vi "CALC_Phi_theta_etc_3_(online).vi"(2 "Current frame #":u32, 3 "Twisted neck":bool, 4 "Use alternative magnets orientation":bool, 5 "Bridge swap":bool, 6 "SB size":u8, 7 "Input cluster of data":T1) -> (1 "Animal coordinates":T2)   [LabVIEW 2018, in "Tracker.lvlib"]
uses:
  Tracker.lvlib
  Controls/CTL_Animal_Coordinates_and_Speed.ctl
  Controls/CTL_Cage_Coords.ctl
  <vilib>/ptbypt/NI_PtbyPt.lvlib
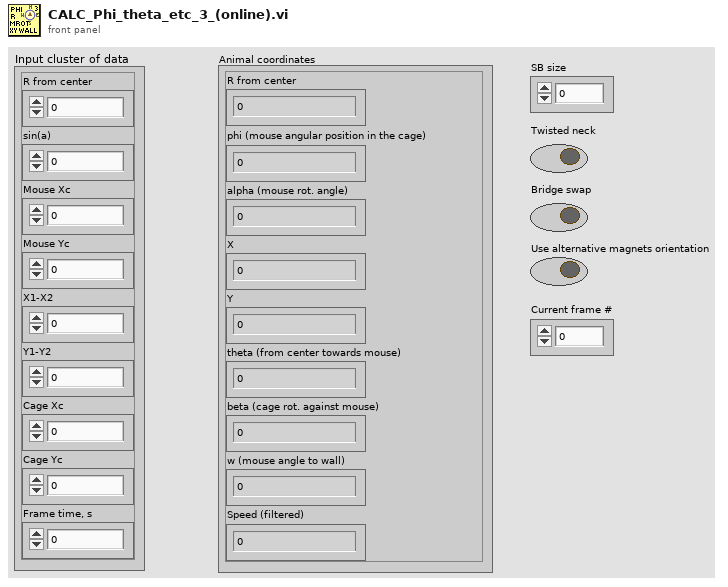
[diagram p1: front panel]
types:
  T1 = typedef "Tracker.lvlib/CTL_Cage_Coords.ctl" = cluster{"R from center":dbl, "sin(a)":dbl, "Mouse Xc":dbl, "Mouse Yc":dbl, "X1-X2":dbl, "Y1-Y2":dbl, "Cage Xc":dbl, "Cage Yc":dbl, "Frame time, s":dbl}
  T2 = typedef "Tracker.lvlib/CTL_Animal_Coordinates_and_Speed.ctl" = cluster{"R from center":dbl, "phi (mouse angular position in the cage)":dbl, "alpha (mouse rot. angle)":dbl, "X":dbl, "Y":dbl, "theta (from center towards mouse)":dbl, "beta (cage rot. against mouse)":dbl, "w (mouse angle to wall)":dbl, "Speed (filtered)":dbl}
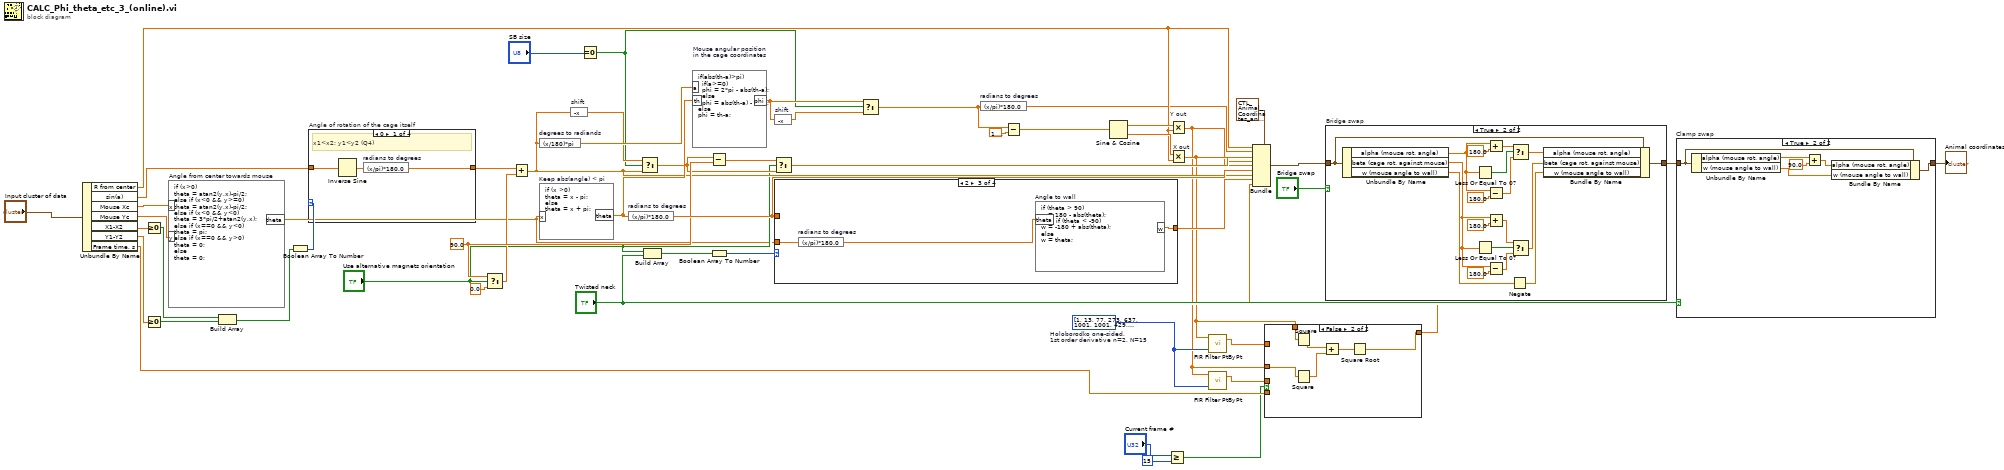
[diagram p0: block diagram]
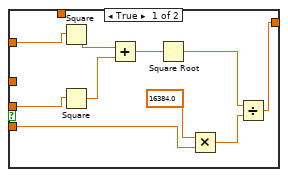
[diagram p2: hidden frame]
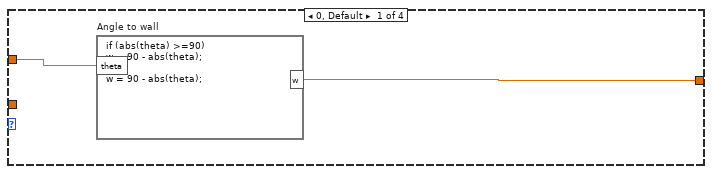
[diagram p4: hidden frame]
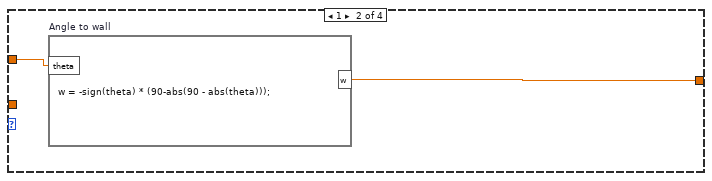
[diagram p5: hidden frame]
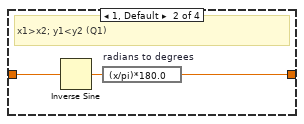
[diagram p8: hidden frame]
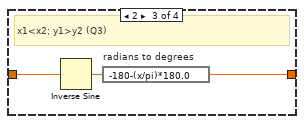
[diagram p9: hidden frame]
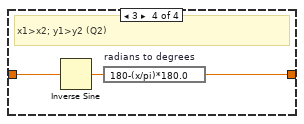
[diagram p10: hidden frame]
diagram:
  w10 = i32[] [1, 13, 77, 273, 637, 1001, 1001, 429, -429, -1001, -1001, -637, -273, -77, -13, -1]  # Holoborodko one-sided, 1st order derivative n=2, N=15
  w28 = 90.0 ("y")
  n1 = Unbundle By Name("Input cluster of data") -> ("R from center"=w37:dbl, "sin(a)"=w42:dbl, "Mouse Xc"=w41:dbl, "Mouse Yc"=w40:dbl, "X1-X2"=w39:dbl, "Y1-Y2"=w38:dbl, "Frame time, s"=w9:dbl)
  n2 = Greater Or Equal To 0?(x=w39) -> (x >= 0?=w54:bool)
  n3 = Greater Or Equal To 0?(x=w38) -> (x >= 0?=w53:bool)
  n4 = formula code="if (x>0)\ntheta = atan2(y,x)-pi/2;\nelse if (x<0 && y>=0)\ntheta = atan2(y,x)-pi/2;\nelse if (x<0 && y<0)\ntheta = 3*pi/2+atan2(y,x);\nelse if (x==0 && y<0)\ntheta = pi;\nelse if (x==0 && y>0)\ntheta = 0;\nelse\ntheta = 0;" "Angle from center towards mouse"("x"=w41, "y"=w40) -> ("theta"=w13:dbl)
  n5 = Build Array(w54, w53) -> (w52:bool[])
  n6 = Boolean Array To Number(Boolean array=w52) -> (number=w51:u32)
  n7 = case "Angle of rotation of the cage itself" shown="0" w51 {
    tunnel: w42 -> [w56 w59 w62 w65]
    tunnel: [w55 w58 w61 w64] -> w31
    frame 0 {
      # "x1<x2; y1<y2 (Q4)"
      n8 = Inverse Sine(1:w56) -> (0:w57:dbl)
      n9 = expression code="(x/pi)*180.0" "radians to degrees"(w57) -> (w55:dbl)
    }
    frame 1, Default {
      # "x1>x2; y1<y2 (Q1)"
      n10 = Inverse Sine(1:w59) -> (0:w60:dbl)
      n11 = expression code="(x/pi)*180.0" "radians to degrees"(w60) -> (w58:dbl)
    }
    frame 2 {
      # "x1<x2; y1>y2 (Q3)"
      n12 = Inverse Sine(1:w62) -> (0:w63:dbl)
      n13 = expression code="-180-(x/pi)*180.0" "radians to degrees"(w63) -> (w61:dbl)
    }
    frame 3 {
      # "x1>x2; y1>y2 (Q2)"
      n14 = Inverse Sine(1:w65) -> (0:w66:dbl)
      n15 = expression code="180-(x/pi)*180.0" "radians to degrees"(w66) -> (w64:dbl)
    }
  }
  n16 = Select(t=w28, s="Use alternative magnets orientation", f=0.0) -> (s? t:f=w27:dbl)
  n17 = Add(x=w31, y=w27) -> (x+y=w25:dbl)
  n18 = expression code="(x/180)*pi" "degrees to radiands"(w25) -> (w47:dbl)
  n19 = formula code="if (x >0)\ntheta = x - pi;\nelse\ntheta = x + pi;" "Keep abs(angle) < pi"("x"=w13) -> ("theta"=w48:dbl)
  n20 = expression code="-x" "shift"(w25) -> (w24:dbl)
  n21 = Equal To 0?(x="SB size") -> (x = 0?=w11:bool)
  n22 = expression code="(x/pi)*180.0" "radians to degrees"(w48) -> (w44:dbl)
  n23 = Select(t=w24, s=w11, f=w25) -> (s? t:f=w26:dbl)
  n24 = Build Array("Use alternative magnets orientation", "Twisted neck") -> (w15:bool[])
  n25 = formula code="if(abs(th-a)>pi)\n  if(a>=0)\n  phi = 2*pi - abs(th-a);\n  else\n  phi = abs(th-a) - 2*pi;\nelse\nphi = th-a;" "Mouse angular position in the cage coordinates"("th"=w48, "a"=w47) -> ("phi"=w22:dbl)
  n26 = Subtract(x=w26, y=w28) -> (x-y=w29:dbl)
  n27 = Boolean Array To Number(Boolean array=w15) -> (number=w14:u32)
  n28 = Select(t=w29, s="Use alternative magnets orientation", f=w26) -> (s? t:f=w30:dbl)
  n29 = expression code="-x" "shift"(w22) -> (w21:dbl)
  n30 = case shown="2" w14 {
    tunnel: w44 -> [w68 w70 _ w74]
    tunnel: [w67 w69 w73 w74] -> w18
    tunnel: w13 -> [_ _ w72 _]
    frame 0, Default {
      n31 = formula code="if (abs(theta) >=90)\nw = 90 - abs(theta);\nelse\nw = 90 - abs(theta);" "Angle to wall"("theta"=w68) -> ("w"=w67:dbl)
    }
    frame 1 {
      n32 = formula code="w = -sign(theta) * (90-abs(90 - abs(theta)));" "Angle to wall"("theta"=w70) -> ("w"=w69:dbl)
    }
    frame 2 {
      n33 = expression code="(x/pi)*180.0" "radians to degrees"(w72) -> (w71:dbl)
      n34 = formula code="if (theta > 90)\nw = 180 - abs(theta);\nelse if (theta < -90)\nw = -180 + abs(theta);\nelse\nw = theta;" "Angle to wall"("theta"=w71) -> ("w"=w73:dbl)
    }
    frame 3 {
    }
  }
  n35 = Select(t=w22, s=w11, f=w21) -> (s? t:f=w23:dbl)
  n36 = expression code="(x/pi)*180.0" "radians to degrees"(w23) -> (w36:dbl)
  n37 = Subtract(x=w23, y=1.5707963267948966) -> (x-y=w46:dbl)
  n38 = Sine & Cosine(0:w46) -> (1:w49:dbl, 2:w50:dbl)
  n39 = Greater Or Equal?(x="Current frame #", y=u32 15) -> (x >= y?=w3:bool)
  n40 = Multiply "Y out"(x=w49, y=w37) -> (x*y=w1:dbl)
  n41 = Multiply "X out"(x=w50, y=w37) -> (x*y=w2:dbl)
  n42 = call <vilib>:"FIR Filter PtByPt.vi"("Forward Coefficients"=w10, "x"=w2) -> ("Filtered x"=w5:dbl)  [unwired: 2 in, 1 out]
  n43 = call <vilib>:"FIR Filter PtByPt.vi"("Forward Coefficients"=w10, "x"=w1) -> ("Filtered x"=w4:dbl)  [unwired: 2 in, 1 out]
  n44 = case shown="False" w3 {
    tunnel: w9 -> [w81 _]
    tunnel: [w80 w87] -> w8
    tunnel: w5 -> [w76 _]
    tunnel: w4 -> [w75 _]
    tunnel: w2 -> [_ w86]
    tunnel: w1 -> [_ w85]
    frame True {
      n45 = Square(x=w76) -> (x^2=w84:dbl)
      n46 = Square(x=w75) -> (x^2=w83:dbl)
      n47 = Add(x=w84, y=w83) -> (x+y=w82:dbl)
      n48 = Square Root(x=w82) -> (sqrt(x)=w78:dbl)
      n49 = Multiply(x=16384.0 ("y"), y=w81) -> (x*y=w77:dbl)
      n50 = Divide(x=w78, y=w77) -> (x/y=w80:dbl)
    }
    frame False {
      n51 = Square(x=w86) -> (x^2=w90:dbl)
      n52 = Square(x=w85) -> (x^2=w89:dbl)
      n53 = Add(x=w90, y=w89) -> (x+y=w88:dbl)
      n54 = Square Root(x=w88) -> (sqrt(x)=w87:dbl)
    }
  }
  n55 = Bundle(cluster=T2 {"R from center"=0.0, "phi (mouse angular position in the cage)"=0.0, "alpha (mouse rot. angle)"=0.0, "X"=0.0, "Y"=0.0, "theta (from center towards mouse)"=0.0, "beta (cage rot. against mouse)"=0.0, "w (mouse angle to wall)"=0.0, "Speed (filtered)"=0.0} ("Output data cluster 2"), "R from center"=w37, "phi (mouse angular position in the cage)"=w36, "alpha (mouse rot. angle)"=w30, "X"=w2, "Y"=w1, "theta (from center towards mouse)"=w44, "beta (cage rot. against mouse)"=w25, "w (mouse angle to wall)"=w18, "Speed (filtered)"=w8) -> (w33:T2)
  n56 = case "Bridge swap" shown="True" "Bridge swap" {
    tunnel: [w91 w103] -> w20
    tunnel: w33 -> [w91 w104]
    frame False {
    }
    frame True {
      n57 = Unbundle By Name(w104) -> ("alpha (mouse rot. angle)"=w102:dbl, "beta (cage rot. against mouse)"=w95:dbl, "w (mouse angle to wall)"=w93:dbl)
      n58 = Less Or Equal To 0?(x=w102) -> (x <= 0?=w109:bool)
      n59 = Less Or Equal To 0?(x=w95) -> (x <= 0?=w96:bool)
      n60 = Add(x=w102, y=sgl 180.0) -> (x+y=w106:dbl)
      n61 = Subtract(x=w102, y=sgl 180.0) -> (x-y=w108:dbl)
      n62 = Add(x=w95, y=sgl 180.0) -> (x+y=w99:dbl)
      n63 = Subtract(x=w95, y=sgl 180.0) -> (x-y=w97:dbl)
      n64 = Negate(x=w93) -> (-x=w92:dbl)
      n65 = Select(t=w106, s=w109, f=w108) -> (s? t:f=w101:dbl)
      n66 = Select(t=w99, s=w96, f=w97) -> (s? t:f=w94:dbl)
      n67 = Bundle By Name(cluster=w104, "alpha (mouse rot. angle)"=w101, "beta (cage rot. against mouse)"=w94, "w (mouse angle to wall)"=w92) -> (w103:T2)
    }
  }
  n68 = case "Clamp swap" shown="True" "Twisted neck" {
    tunnel: [w110 w114] -> w19
    tunnel: w20 -> [w110 w115]
    frame False {
    }
    frame True {
      n69 = Unbundle By Name(w115) -> ("alpha (mouse rot. angle)"=w113:dbl, "w (mouse angle to wall)"=w112:dbl)
      n70 = Add(x=w113, y=sgl 90.0) -> (x+y=w111:dbl)
      n71 = Bundle By Name(cluster=w115, "alpha (mouse rot. angle)"=w111, "w (mouse angle to wall)"=w112) -> (w114:T2)
    }
  }
  "Animal coordinates" <- w19
